vi "Untitled 2.vi"() -> ()   [LabVIEW 2015]
panel:
  out "data value":i32[][](array[numeric])
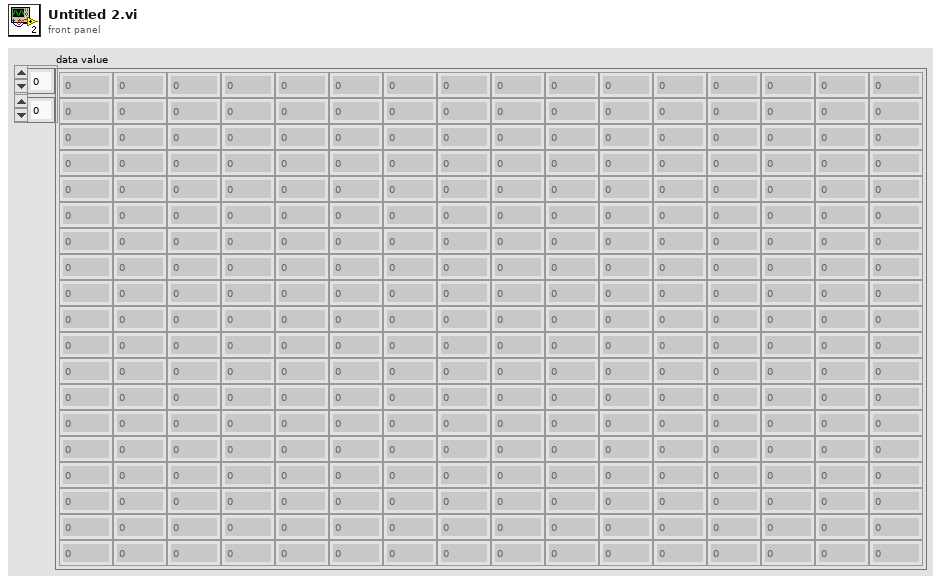
[diagram p1: front panel]
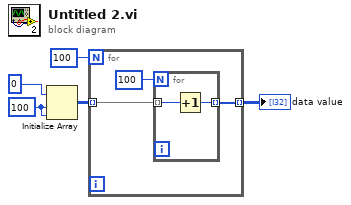
[diagram p0: block diagram]
diagram:
  w4 = 100 ("dimension size")
  n1 = Initialize Array(0, w4, w4) -> (w1:i32[][])
  n2 = for {
    N: 100 ("dimension size") -> [_]
    tunnel: w1 -> [w8] mode=indexing
    tunnel: [w7] -> w3 mode=indexing
    n3 = for {
      N: 100 ("dimension size") -> [_]
      tunnel: w8 -> [w10] mode=indexing
      tunnel: [w9] -> w7 mode=indexing
      n4 = Increment(x=w10) -> (x+1=w9:i32)
    }
  }
  "data value" <- w3
